vi "Create Mask.vi"(8 "Error in":errorcluster caption="Error in (no error)", 11 "Mask In":refnum<class "Mask.lvclass">) -> (0 "Error out":errorcluster, 3 "Mask Out":refnum<class "Mask.lvclass">)   [LabVIEW 2016, in "Mask.lvclass"]
uses:
  Mask.lvclass
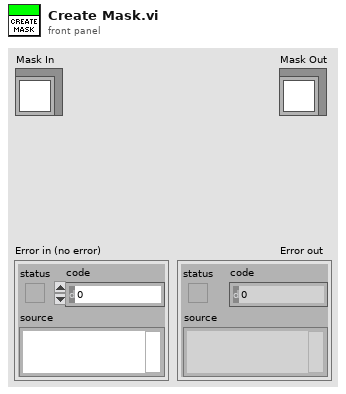
[diagram p1: front panel]
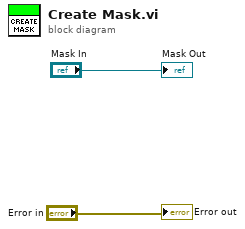
[diagram p0: block diagram]
diagram:
  "Error out" <- "Error in"
  "Mask Out" <- "Mask In"
